vi "Has Events.vi"(8 "error in (no error)":errorcluster, 11 "JKI SM in":refnum<class "JKI SM.lvclass">) -> (0 "error out":errorcluster, 2 "Registered for Events?":bool, 3 "JKI SM out":refnum<class "JKI SM.lvclass">)   [LabVIEW 2020, in "JKI State Machine API.lvlib" / "JKI SM.lvclass"]
uses:
  JKI SM.lvclass
  JKI SM.lvclass/JKI SM.ctl
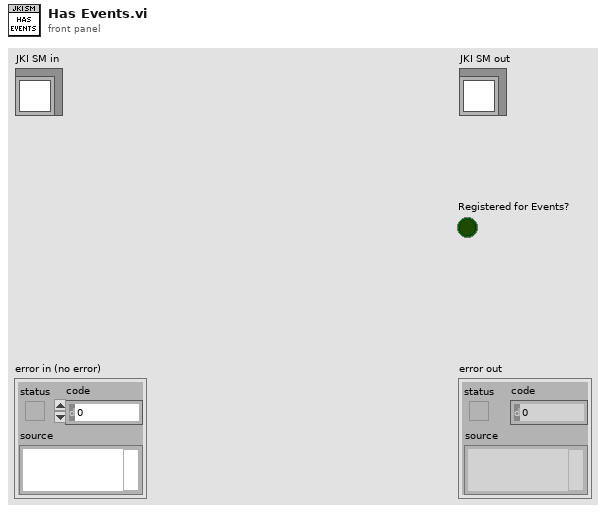
[diagram p1: front panel]
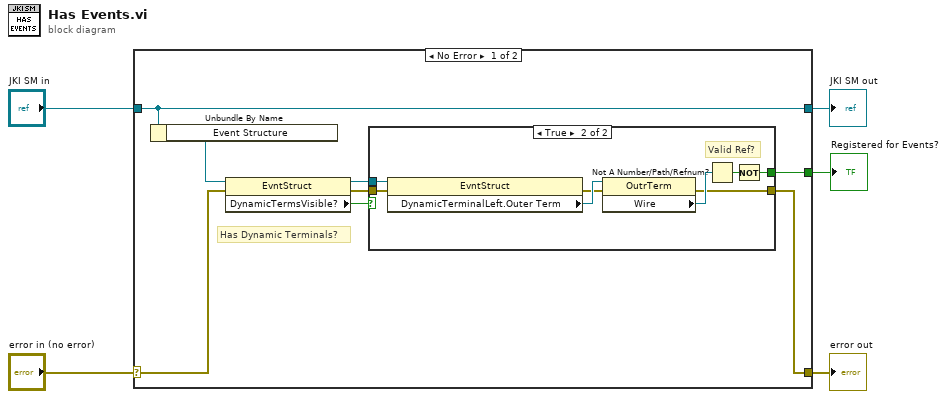
[diagram p0: block diagram]
diagram:
  n1 = case shown="No Error" "error in (no error)" {
    selector: "error in (no error)" -> [w6 w24]
    tunnel: [w7 w24] -> w4
    tunnel: [w13 w23] -> w2
    tunnel: "JKI SM in" -> [w13 w23]
    tunnel: [w9 _] -> w1
    frame No Error {
      # "Has Dynamic Terminals?"
      n2 = Unbundle By Name(w13) -> ("Event Structure"=w12:refnum<vi>)
      n3 = property class="EvntStruct"(reference=w12, error in=w6) -> (reference out=w10:refnum<vi>, error out=w8:errorcluster, "DynamicTermsVisible?"=w11:bool)
      n4 = case shown="True" w11 {
        tunnel: w10 -> [_ w22]
        tunnel: [_ w18] -> w9
        tunnel: w8 -> [w14 w17]
        tunnel: [w14 w15] -> w7
        frame False {
        }
        frame True {
          # "Valid Ref?"
          n5 = property class="EvntStruct"(reference=w22, error in=w17) -> (error out=w16:errorcluster, "DynamicTerminalLeft.Outer Term"=w21:refnum<vi>)  [unwired: 1 out]
          n6 = property class="OutrTerm"(reference=w21, error in=w16) -> (error out=w15:errorcluster, "Wire"=w20:refnum<vi>)  [unwired: 1 out]
          n7 = Not A Number/Path/Refnum?(number/path/refnum=w20) -> (NaN/Path/Refnum?=w19:bool)
          n8 = Not(x=w19) -> (.not. x?=w18:bool)
        }
      }
    }
    frame Error {
    }
  }
  "error out" <- w4
  "JKI SM out" <- w2
  "Registered for Events?" <- w1
